vi "未命名 2.vi"() -> ()   [LabVIEW 2020]
panel:
  out "工位1_数据表显示":string[][](table)
  out "实时压力(MPa/S）":dbl
  out "爆破速率(MPa/S)":dbl
  out "爆破压力(MPa)":dbl
  out "上保压时间(S)":i32
  out "上呼吸速率(MPa/S)":dbl
  out "上呼吸压力(MPa)":dbl
  out "下保压时间(S)":i32
  out "下呼吸速率(MPa/S)":dbl
  out "下呼吸压力(MPa)":dbl
  out "呼吸破裂标识":i32
  out "呼吸剩余次数":i32
  out "呼吸循环次数":i32
  out "工位号":i32
  out "运行标志":i32
  out "型号规格":string
  out "连接的字符串":string
  in  "停止":bool
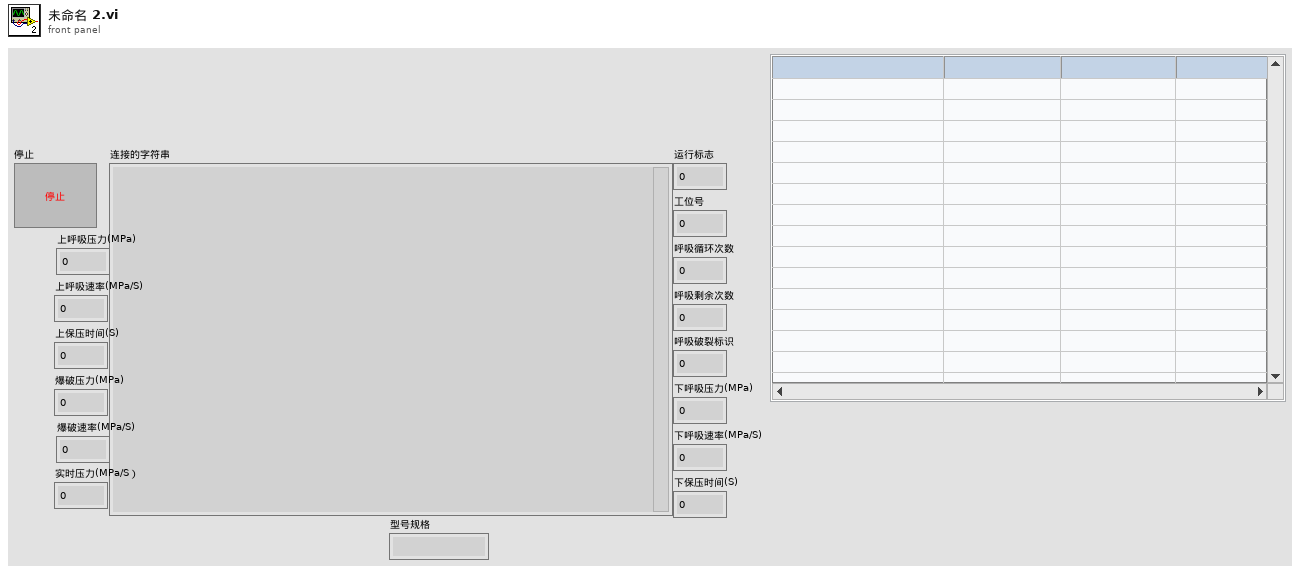
[diagram p1: front panel]
types:
  T1 = enum16{"Standard", "Buffered", "CRLF", "Immediate"}
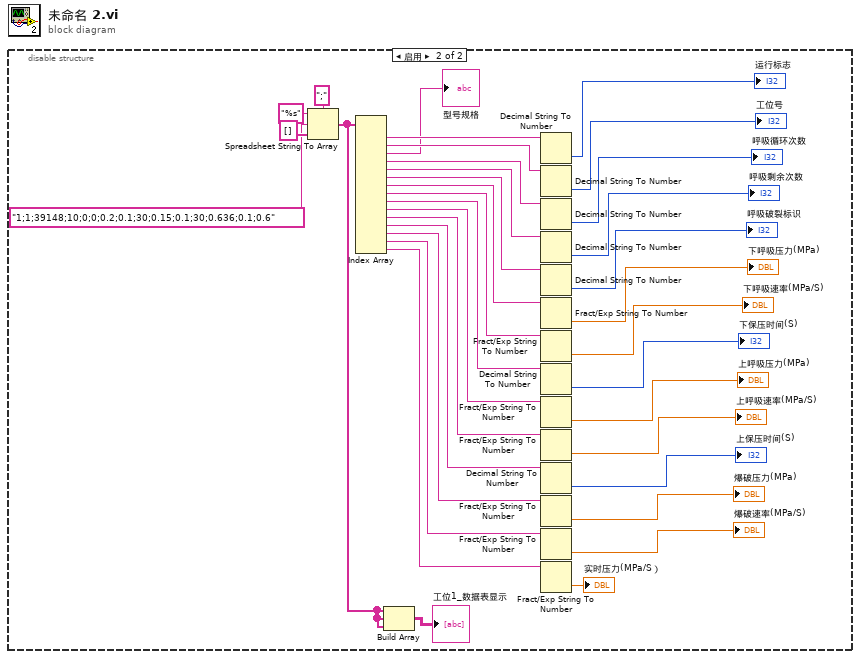
[diagram p0: block diagram]
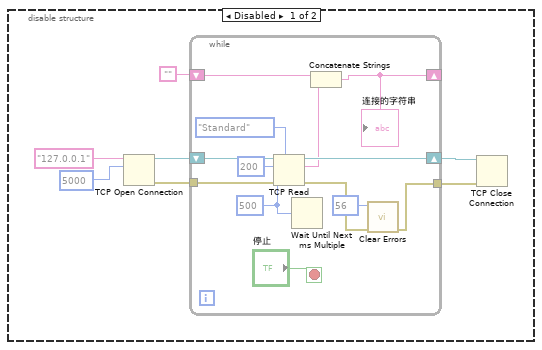
[diagram p2: hidden frame]
diagram:
  n1 = disable-structure shown="启用" {
    frame Disabled {
      n2 = TCP Open Connection(address="127.0.0.1" ("地址"), remote port or service name=u16 5000 ("远程端口或服务名称")) -> (connection ID=w5:refnum<k5>, error out=w2:errorcluster)  [unwired: 3 in]
      n3 = while {
        shift-right: [w16] -> w4
        shift-left: w5 -> [w19]
        shift-right: [w12] -> _
        shift-left: "" -> [w14]
        tunnel: w2 -> [w9]
        tunnel: [w8] -> w1
        stop <- "停止" stop-if-true
        w15 = 500 ("超时毫秒(25000)")
        n4 = TCP Read(connection ID=w19, bytes to read=200 ("读取的字节"), error in (no error)=w9, 7:T1."Standard" ("模式（标准）"), 9:w15) -> (connection ID out=w16:refnum<k5>, data out=w13:string, error out=w11:errorcluster)
        n5 = Wait Until Next ms Multiple(millisecond multiple=w15) -> ()  [unwired: 1 out]
        n6 = Concatenate Strings(w14, w13) -> (w12:string)
        "连接的字符串" <- w12
        n7 = call <vilib>:"Clear Errors.vi"("error in (no error)"=w11, "specific error code to clear (0: all)"=56) -> ("error out"=w8:errorcluster)  [unwired: 4 in, 1 out]
      }
      n8 = TCP Close Connection(connection ID=w4, error in (no error)=w1) -> ()  [unwired: 1 in, 2 out]
    }
    frame Enabled {
      n9 = Spreadsheet String To Array(delimiter (Tab)=";" ("分隔符(Tab)"), format string="%s" ("格式字符串"), spreadsheet string="1;1;39148;10;0;0;0.2;0.1;30;0.15;0.1;30;0.636;0.1;0.6", array type (2D Dbl)=string[] []) -> (array=w22:string[])
      n10 = Index Array(array=w22) -> (element #1=w52:string, element #2=w51:string, element #3=→"型号规格":string, element #4=w50:string, element #5=w49:string, element #6=w48:string, element #7=w47:string, element #8=w46:string, element #9=w45:string, element #10=w44:string, element #11=w43:string, element #12=w42:string, element #13=w41:string, element #14=w40:string, element #15=w39:string)  [unwired: 15 in]
      n11 = Build Array(w22, w22, w22) -> (→"工位1_数据表显示":string[][])
      n12 = Decimal String To Number(string=w52) -> (number=→"运行标志":i32)  [unwired: 2 in, 1 out]
      n13 = Decimal String To Number(string=w51) -> (number=→"工位号":i32)  [unwired: 2 in, 1 out]
      n14 = Decimal String To Number(string=w50) -> (number=→"呼吸循环次数":i32)  [unwired: 2 in, 1 out]
      n15 = Decimal String To Number(string=w49) -> (number=→"呼吸剩余次数":i32)  [unwired: 2 in, 1 out]
      n16 = Decimal String To Number(string=w48) -> (number=→"呼吸破裂标识":i32)  [unwired: 2 in, 1 out]
      n17 = Fract/Exp String To Number(string=w47) -> (number=→"下呼吸压力(MPa)":dbl)  [unwired: 3 in, 1 out]
      n18 = Fract/Exp String To Number(string=w46) -> (number=→"下呼吸速率(MPa/S)":dbl)  [unwired: 3 in, 1 out]
      n19 = Decimal String To Number(string=w45) -> (number=→"下保压时间(S)":i32)  [unwired: 2 in, 1 out]
      n20 = Fract/Exp String To Number(string=w44) -> (number=→"上呼吸压力(MPa)":dbl)  [unwired: 3 in, 1 out]
      n21 = Fract/Exp String To Number(string=w43) -> (number=→"上呼吸速率(MPa/S)":dbl)  [unwired: 3 in, 1 out]
      n22 = Decimal String To Number(string=w42) -> (number=→"上保压时间(S)":i32)  [unwired: 2 in, 1 out]
      n23 = Fract/Exp String To Number(string=w41) -> (number=→"爆破压力(MPa)":dbl)  [unwired: 3 in, 1 out]
      n24 = Fract/Exp String To Number(string=w40) -> (number=→"爆破速率(MPa/S)":dbl)  [unwired: 3 in, 1 out]
      n25 = Fract/Exp String To Number(string=w39) -> (number=→"实时压力(MPa/S）":dbl)  [unwired: 3 in, 1 out]
    }
  }
